vi "Hanning Window (DBL).vi"(0 "X":dbl[](array[numeric])) -> (1 "Windowed X":dbl[](array[numeric]), 2 "error":i32)   [LabVIEW 2024, in "NI_AALPro.lvlib"]
doc: "<p>Applies a Hanning window to the input signal <strong>X</strong>. Wire data to the <strong>X</strong> input to determine the polymorphic instance to use or <a href=\"nihelplauncher://docs/csh?context=lvcore_lvhowto_selectingdefaultinstpolyvi\">manually select</a> the instance.</p>"
uses:
  NI_AALPro.lvlib
panel:
  # "Hanning Window"
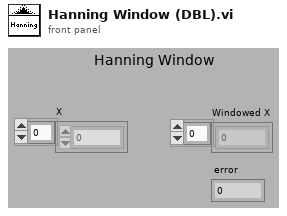
[diagram p1: front panel]
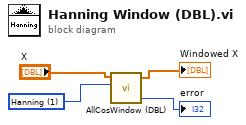
[diagram p0: block diagram]
diagram:
  w3 = u16 1 items=["None "=0, "Hanning"=1, "Hamming"=2, "Blackman-Harris"=3, "Exact Blackman"=4, "Blackman"=5, "Flat Top"=6, "4 Term B-Harris "=7, "7 Term B-Harris"=8, "Low Sidelobe"=9, "Blackman Nuttall"=14] ("window")
  n1 = call "AllCosWindow (DBL).vi"("window"=w3, "X"="X") -> ("error"=→"error":i32, "Windowed X"=→"Windowed X":dbl[])  [unwired: 3 in]
